vi "Plot Colors.vi"(11 "Plot Index":i32) -> (3 "Color Box":u32(colorbox)=6618880)   [LabVIEW 2021, in "RocketPlot.lvlib"]
uses:
  RocketPlot.lvlib
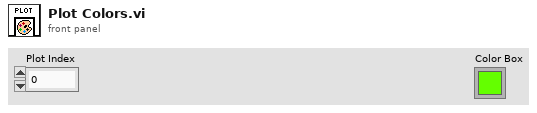
[diagram p1: front panel]
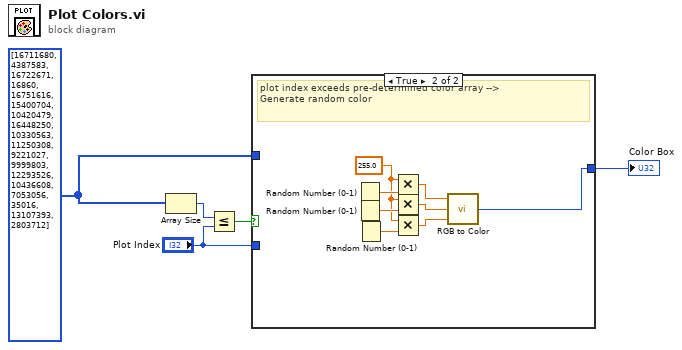
[diagram p0: block diagram]
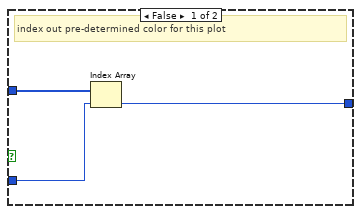
[diagram p2: hidden frame]
diagram:
  w3 = u32[] [16711680, 4387583, 16722671, 16860, 16751616, 15400704, 10420479, 16448250, 10330563, 11250308, 9221027, 9999803, 12293526, 10436608, 7053056, 35016, 13107393, 2803712]
  n1 = Array Size(array=w3) -> (size(s)=w4:i32)
  n2 = Less Or Equal?(x=w4, y="Plot Index") -> (x <= y?=w5:bool)
  n3 = case shown="True" w5 {
    tunnel: w3 -> [w8 _]
    tunnel: "Plot Index" -> [w7 _]
    tunnel: [w6 w16] -> w1
    frame False {
      # "index out pre-determined color for this plot"
      n4 = Index Array(array=w8, index=w7) -> (element=w6:u32)
    }
    frame True {
      w12 = 255.0 ("x")
      # "plot index exceeds pre-determined color array -->\nGenerate random color"
      n5 = Random Number (0-1)() -> (number: 0 to 1=w15:dbl)
      n6 = Random Number (0-1)() -> (number: 0 to 1=w13:dbl)
      n7 = Random Number (0-1)() -> (number: 0 to 1=w14:dbl)
      n8 = Multiply(x=w12, y=w15) -> (x*y=w11:dbl)
      n9 = Multiply(x=w12, y=w13) -> (x*y=w10:dbl)
      n10 = Multiply(x=w12, y=w14) -> (x*y=w9:dbl)
      n11 = call <vilib>:"RGB to Color.vi"("B"=w9, "G"=w10, "R"=w11) -> ("Color"=w16:u32)
    }
  }
  "Color Box" <- w1
